vi "Send_Billede-Steffen’s MacBook Pro.vi"() -> ()   [LabVIEW 2018]
uses:
  <vilib>/myRIO/Instrument Drivers/Onboard IO/UART/typedef/VISA Configuration.ctl
  <vilib>/Instr/_visa.llb/VISA Configure Serial Port (Instr).vi
  <vilib>/myRIO/Express VI/Onboard IO/UART/UART Express VI.xnode
  <vilib>/myRIO/Instrument Drivers/Onboard IO/UART/UART.lvlib
panel:
  out "element":i32
  out "output array":i32[](array[numeric])
  out "appended array 3":i32[](array[numeric])
  out "appended array 2":i32[](array[numeric])
  out "length":i32
  out "spreadsheet string":string
  out "Subarray":i32
  out "size(s)":i32[](array[numeric])
  out "Intensity Graph 5":u8[][](graph)
  out "Intensity Graph 4":u8[][](graph)
  out "appended array":u8[][](array[numeric])
  out "subarray":u8[](array[numeric])
  out "element 2":i32
  out "array":u8[][](array[numeric])
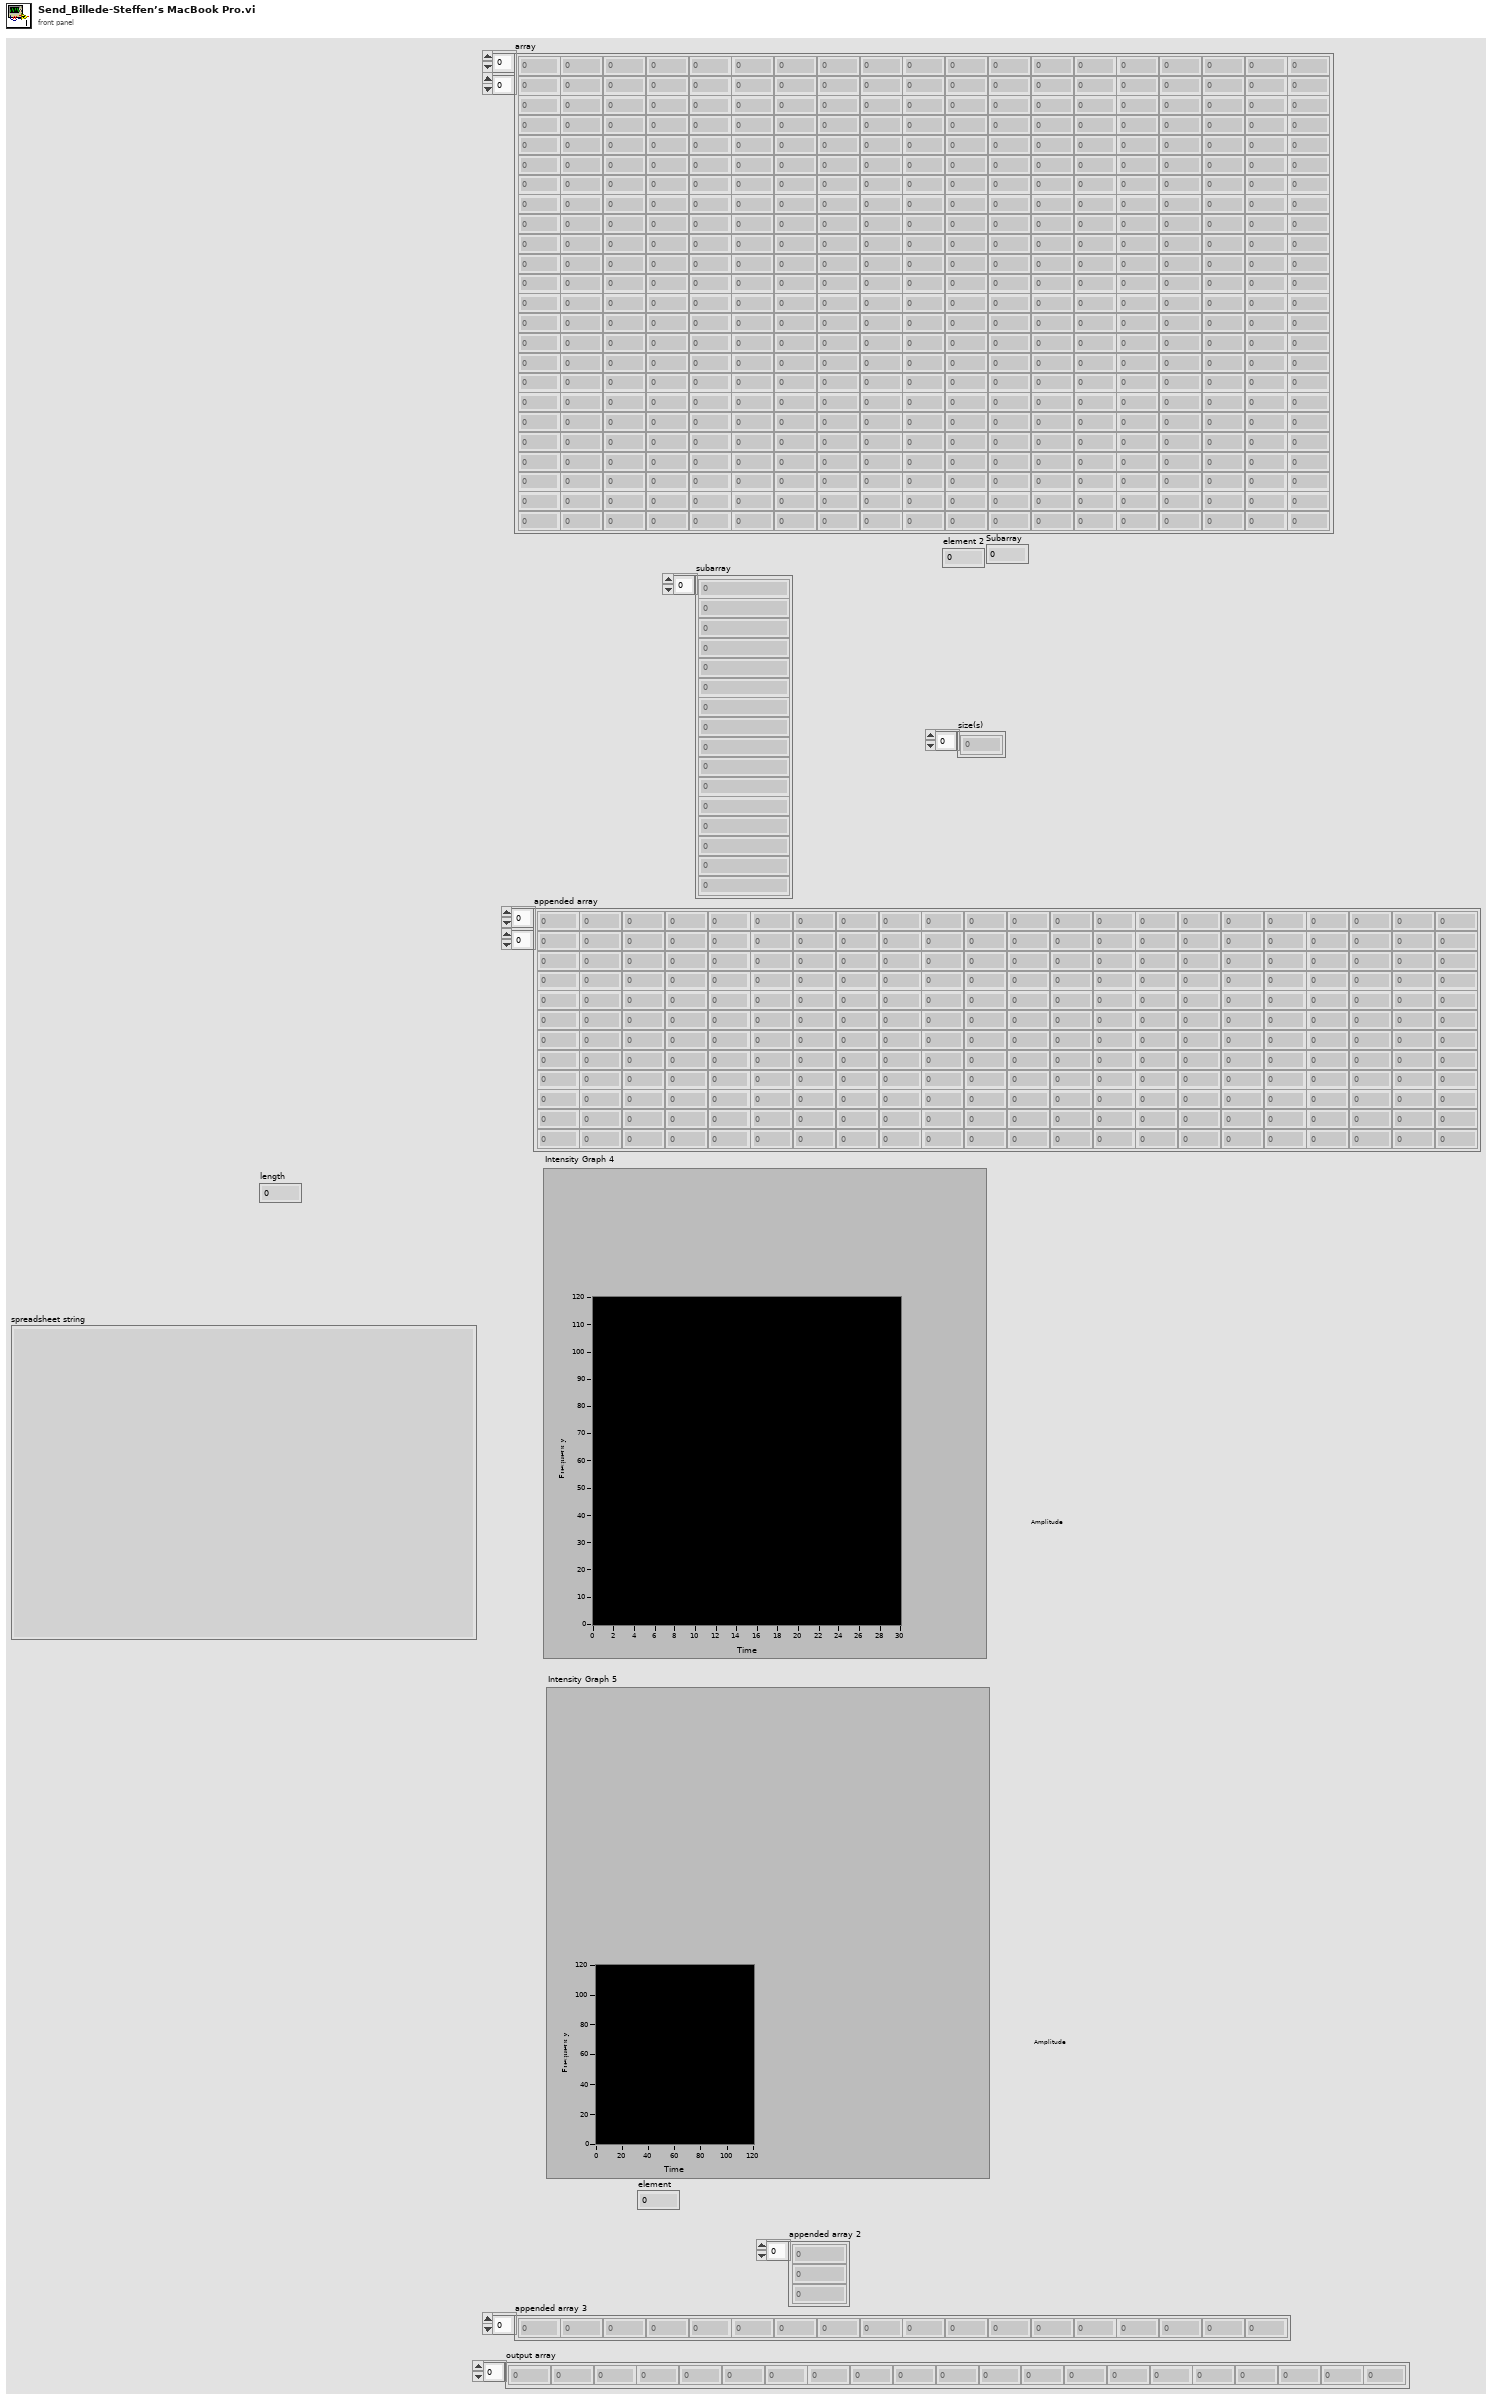
[diagram p1: front panel]
types:
  T1 = typedef "UART.lvlib/VISA Configuration.ctl" = cluster{"baud rate (9600)":u32, "data bits (8)":u16, "parity (0:none)":enum16{"None", "Odd", "Even", "Mark", "Space"}, "stop bits (10: 1 bit)":u16, "flow control (0:none)":u16, "termination char\n(0xA = '\\n' = LF) ":u8, "Enable Termination\nChar (T)":bool, "timeout (10sec)":u32}
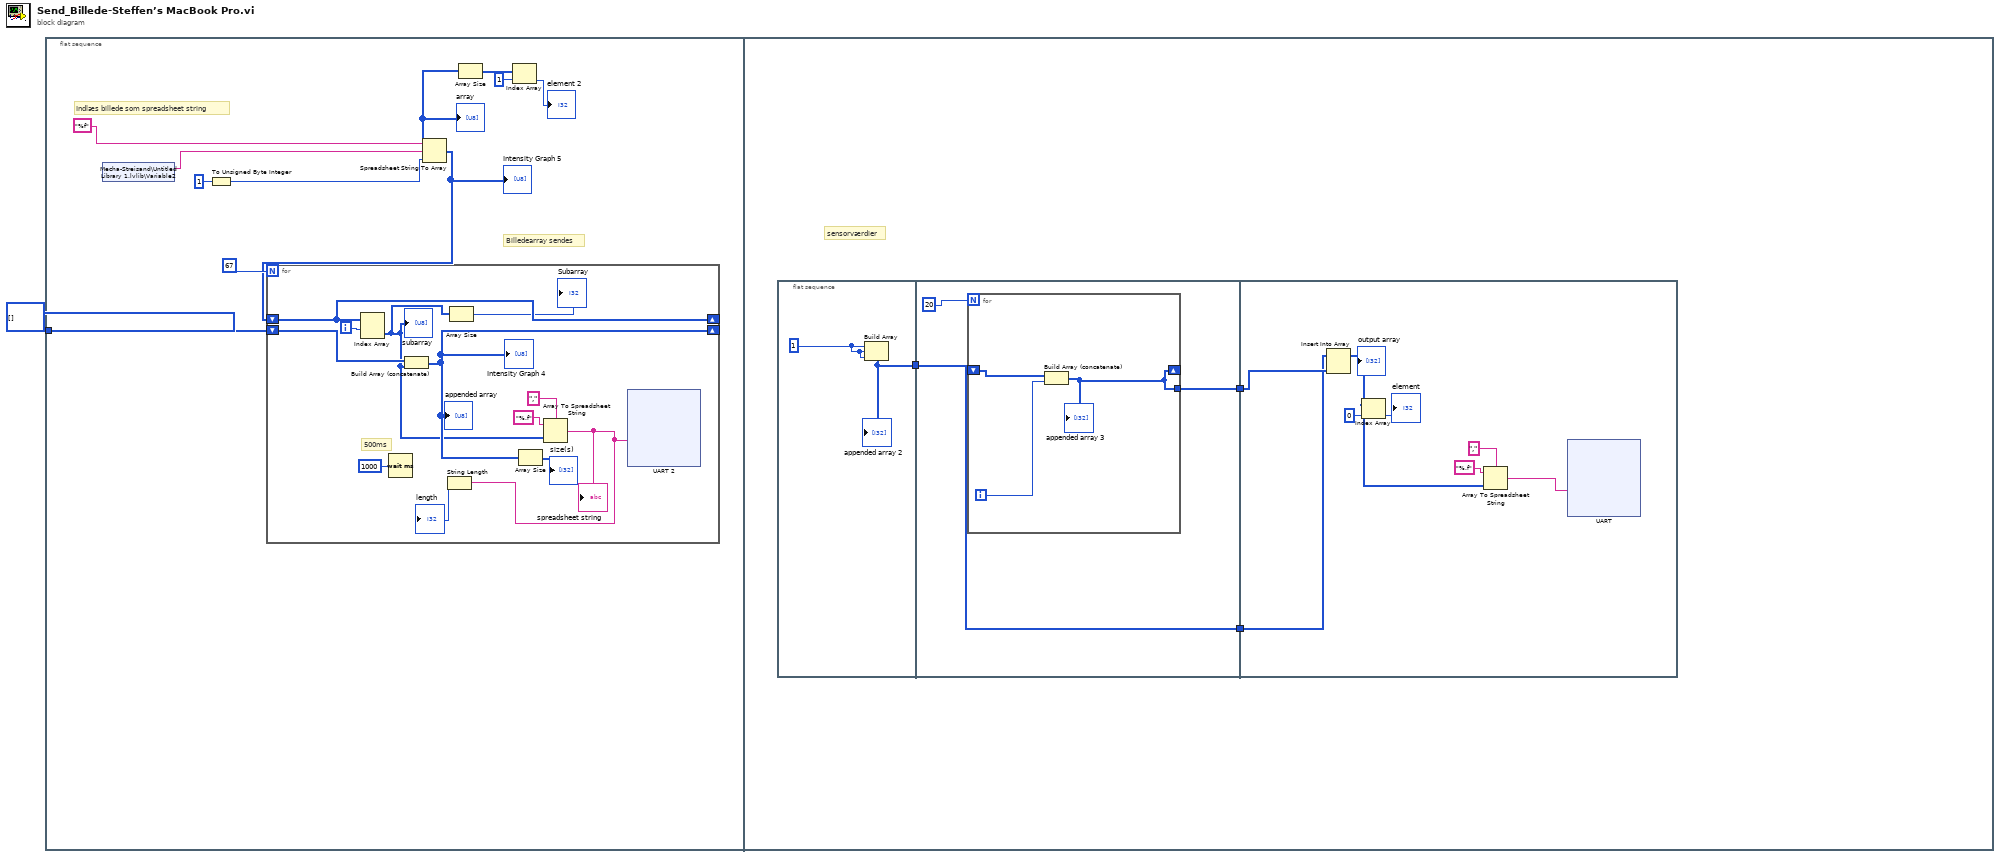
[diagram p0: block diagram]
diagram:
  n1 = flat-sequence {
    tunnel: u8[][] [] -> [w10]
    frame #0 {
      # "Indlæs billede som spreadsheet string"
      # "Billedearray sendes"
      n2 = shared-variable "Mecha-Streisand\\Untitled Library 1.lvlib\\Variable2"() -> (w9:string)  [unwired: 1 in, 1 out]
      n3 = To Unsigned Byte Integer(number=u8 1) -> (unsigned 8bit integer=w6:u8)
      n4 = Spreadsheet String To Array(format string="%f", spreadsheet string=w9, array type (2D Dbl)=w6) -> (array=w2:u8[][])  [unwired: 1 in]
      "array" <- w2
      "Intensity Graph 5" <- w2
      n5 = for {
        N: 67 -> [_]
        shift-right: [w23] -> _
        shift-left: w2 -> [w23]
        shift-right: [w17] -> _
        shift-left: w10 -> [w22]
        i -> [w21]
        # "500ms"
        n6 = Index Array(array=w23, index (row)=w21) -> (element=w14:u8[])  [unwired: 1 in]
        "subarray" <- w14
        n7 = Wait (ms)(milliseconds to wait=u32 1000) -> ()  [unwired: 1 out]
        n8 = Build Array (concatenate)(w22, w14) -> (w17:u8[][])
        "appended array" <- w17
        "Intensity Graph 4" <- w17
        n9 = Array Size(array=w14) -> (size(s)=→"Subarray":i32)
        n10 = Array Size(array=w17) -> (size(s)=→"size(s)":i32[])
        n11 = Array To Spreadsheet String(delimiter (Tab)=",", array=w14, 3:"%.f" ("format string")) -> (spreadsheet string=w13:string)
        "spreadsheet string" <- w13
        n12 = String Length(string=w13) -> (length=→"length":i32)
        n13 = xnode "UART 2"("Characters to Write"=w13) -> ()  [unwired: 1 in, 2 out]
      }
      n14 = Array Size(array=w2) -> (size(s)=w7:i32[])
      n15 = Index Array(array=w7, index=1) -> (element=→"element 2":i32)
    }
    frame #1 {
      # "sensorværdier"
      n16 = flat-sequence {
        tunnel: [w44] -> w41
        tunnel: [w46] -> w42
        tunnel: w41 -> [w46]
        tunnel: [w45] -> w40
        tunnel: w42 -> [w57]
        tunnel: w40 -> [w58]
        frame #0 {
          w43 = 1
          n17 = Build Array(w43, w43, w43) -> (w44:i32[])
          "appended array 2" <- w44
        }
        frame #1 {
          n18 = for {
            N: 20 -> [_]
            shift-right: [w48] -> _
            shift-left: _ -> [w49]
            tunnel: [w48] -> w45
            i -> [w50]
            n19 = Build Array (concatenate)(w49, w50) -> (w48:i32[])
            "appended array 3" <- w48
          }
        }
        frame #2 {
          n20 = Insert Into Array(array=w57, new element=w58) -> (w51:i32[])  [unwired: 1 in]
          "output array" <- w51
          n21 = Index Array(array=w51, index=0) -> (element=→"element":i32)
          n22 = Array To Spreadsheet String(delimiter (Tab)=",", array=w51, 3:"%.f" ("format string")) -> (spreadsheet string=w52:string)
          n23 = xnode "UART"("Characters to Write"=w52) -> ()  [unwired: 1 in, 2 out]
        }
      }
    }
  }
